vi "Rank HV combos.vi"(10 "H Scores":T2(array[cluster]), 11 "Vertical":T3) -> (3 "Target Scores":cluster{dbl, dbl, dbl, dbl, dbl, i32, T1}[](array[cluster]))   [LabVIEW 2014]
uses:
  TargetType.ctl
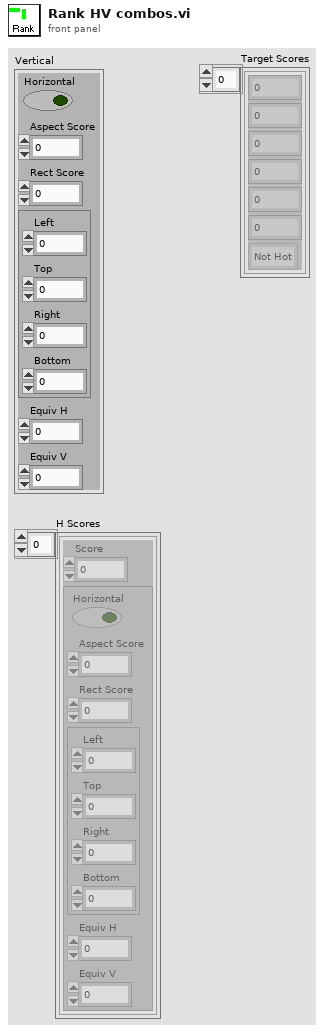
[diagram p1: front panel]
types:
  T1 = typedef "TargetType.ctl" = enum16{"Not Hot", "Hot"}
  T2 = cluster{"Score":dbl, cluster{"Horizontal":bool, "Aspect Score":dbl, "Rect Score":dbl, cluster{"Left":dbl, "Top":dbl, "Right":dbl, "Bottom":dbl}, "Equiv H":dbl, "Equiv V":dbl}}[]
  T3 = cluster{"Horizontal":bool, "Aspect Score":dbl, "Rect Score":dbl, cluster{"Left":dbl, "Top":dbl, "Right":dbl, "Bottom":dbl}, "Equiv H":dbl, "Equiv V":dbl}
  T4 = cluster{"Left":dbl, "Top":dbl, "Right":dbl, "Bottom":dbl}
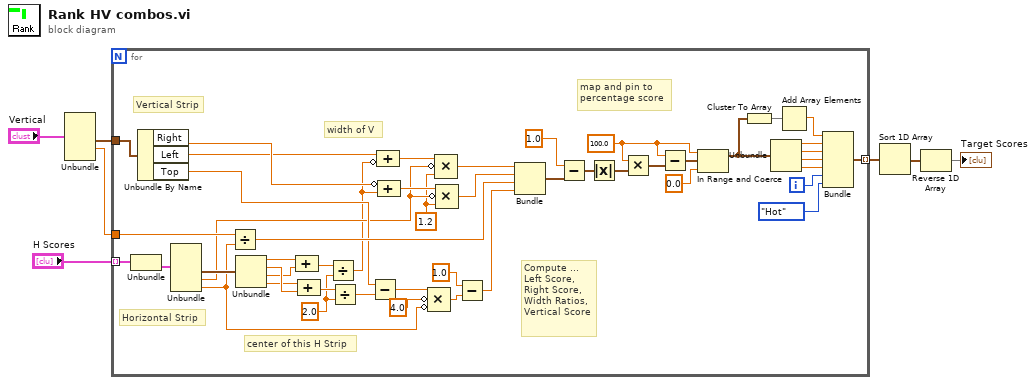
[diagram p0: block diagram]
diagram:
  n1 = Unbundle("Vertical") -> (w1:T4, "Equiv H"=w2:dbl)  [unwired: 4 out]
  n2 = for {
    tunnel: "H Scores" -> [w55] mode=indexing
    tunnel: w1 -> [w54]
    tunnel: [w10] -> w3 mode=indexing
    tunnel: w2 -> [w25]
    i -> [w9]
    w18 = 1.2
    w28 = 100.0 ("x/y")
    w22 = 2.0
    # "Horizontal Strip"
    # "Vertical Strip"
    # "map and pin to\npercentage score"
    # "Compute ...\nLeft Score,\nRight Score,\nWidth Ratios,\nVertical Score"
    # "center of this H Strip"
    # "width of V"
    n3 = Unbundle(w55) -> (w53:T3)  [unwired: 1 out]
    n4 = Unbundle By Name(w54) -> ("Right"=w51:dbl, "Left"=w42:dbl, "Top"=w41:dbl)
    n5 = Unbundle(w53) -> (w52:T4, "Equiv H"=w24:dbl, "Equiv V"=w26:dbl)  [unwired: 3 out]
    n6 = Divide(x=w25, y=w26) -> (x/y=w43:dbl)
    n7 = Unbundle(w52) -> ("Left"=w21:dbl, "Top"=w40:dbl, "Right"=w20:dbl, "Bottom"=w39:dbl)
    n8 = Compound Arithmetic op=ADD(w21, w20) -> (w23:dbl)
    n9 = Compound Arithmetic op=ADD(w39, w40) -> (w50:dbl)
    n10 = Divide(x=w23, y=w22) -> (x/y=w19:dbl)
    n11 = Divide(x=w50, y=w22) -> (x/y=w49:dbl)
    n12 = Subtract(x=w41, y=w49) -> (x-y=w48:dbl)
    n13 = Compound Arithmetic op=ADD(w42, invert w19) -> (w47:dbl)
    n14 = Compound Arithmetic op=ADD(invert w51, w19) -> (w46:dbl)
    n15 = Compound Arithmetic op=MULTIPLY(w48, invert 4.0, invert w26) -> (w38:dbl)
    n16 = Compound Arithmetic op=MULTIPLY(w47, invert w24, w18) -> (w45:dbl)
    n17 = Compound Arithmetic op=MULTIPLY(w46, invert w24, w18) -> (w44:dbl)
    n18 = Subtract(x=1.0, y=w38) -> (x-y=w36:dbl)
    n19 = Bundle(w45, w44, w43, w36) -> (w29:cluster{dbl, dbl, dbl, dbl})  [unwired: 1 in]
    n20 = Subtract(x=1.0 ("y"), y=w29) -> (x-y=w32:cluster{dbl, dbl, dbl, dbl})
    n21 = Absolute Value(x=w32) -> (abs(x)=w34:cluster{dbl, dbl, dbl, dbl})
    n22 = Multiply(x=w28, y=w34) -> (x*y=w35:cluster{dbl, dbl, dbl, dbl})
    n23 = Subtract(x=w28, y=w35) -> (x-y=w31:cluster{dbl, dbl, dbl, dbl})
    n24 = In Range and Coerce(upper limit=w28, x=w31, lower limit=0.0) -> (coerced(x)=w16:cluster{dbl, dbl, dbl, dbl})  [unwired: 1 out]
    n25 = Cluster To Array(cluster=w16) -> (array=w17:dbl[])
    n26 = Unbundle(w16) -> (w12:dbl, w13:dbl, w14:dbl, w15:dbl)
    n27 = Add Array Elements(numeric array=w17) -> (sum=w11:dbl)
    n28 = Bundle(w11, w12, w13, w14, w15, w9, TargetType."Hot") -> (w10:cluster{dbl, dbl, dbl, dbl, dbl, i32, T1})  [unwired: 1 in]
  }
  n29 = Sort 1D Array(array=w3) -> (sorted array=w4:cluster{dbl, dbl, dbl, dbl, dbl, i32, T1}[])
  n30 = Reverse 1D Array(array=w4) -> (reversed array=→"Target Scores":cluster{dbl, dbl, dbl, dbl, dbl, i32, T1}[])
